vi "WaveformDAQ_tb2.vi"() -> ()   [LabVIEW 2018]
uses:
  <vilib>/DAQmx/read.llb/DAQmx Read (Analog Wfm 1Chan NSamp).vi
  <vilib>/DAQmx/create/channels.llb/DAQmx Create Channel (AI-Voltage-Basic).vi
  <vilib>/DAQmx/configure/timing.llb/DAQmx Timing (Sample Clock).vi
  <vilib>/DAQmx/miscellaneous.llb/DAQmx Fill In Error Info.vi
  <instrlib>/Agilent 33XXX Series/Agilent 33XXX Series.lvlib
  <resource>/objmgr/daqmx.rc
panel:
  out "Waveform Graph 2":waveform(dbl)(graph)
  in  "Sample Clock Source":tag="OnboardClock"
  out "error out":errorcluster
  out "Actual Sample Rate":dbl=1000.0 format="%0.2f"
  in  "Sample Mode":i32(ring)=10123 items=["Finite Samples"=10178, "Continuous Samples"=10123, "Hardware Timed Single Point"=12522]
  in  "Terminal Configuration":i32(ring)=-1 items=["default"=-1, "RSE"=10083, "NRSE"=10078, "Differential"=10106, "Pseudodifferential"=12529]
  in  "Voltage Max Value":dbl=5.0 caption="Max Value"
  in  "Voltage Min Value":dbl=-5.0 caption="Min Value"
  in  "Voltage Physical Channels":tag="Dev1/ai0" caption="Physical Channels"
  in  "stop":bool
  out "Waveform Graph":waveform(dbl)(graph)
  in  "Amplitude (1 Vpp)":dbl=1.0
  in  "DC Offset (0.00 V)":dbl
  in  "Waveform Function (1: Sine)":u16(ring)=1 items=["DC", "Sine", "Square", "Triangle", "Ramp", "Pulse", "Noise", "Sinc", "Negative Ramp", "Exponential Rise", "Exponential Fall", "Cardiac"]
  in  "Frequency (1000 Hz)":dbl=1000.0
  in  "Sample rate":enum16{"1KHz", "10KHz", "100KHz", "1MHz"}(ring)
  in  "Time":dbl
  out "N Samples":dbl
  in  "Serial Configuration":T1={"Baud Rate"=9600, "Parity"=0, "Data Bits"=8, "Flow Control"=4} {"Flow Control" items=["None", "XON/XOFF", "RTS/CTS", "XON/XOFF & RTS/CTS", "DTR/DSR", "XON/XOFF & DTR/DSR"]; "Data Bits" items=["7"=7, "8"=8]; "Parity" items=["None", "Odd", "Even", "Mark", "Space"]; "Baud Rate" items=["300"=300, "600"=600, "1200"=1200, "2400"=2400, "4800"=4800, "9600"=9600, "19200"=19200]}
  in  "VISA resource name":refnum<visa-resource-name>
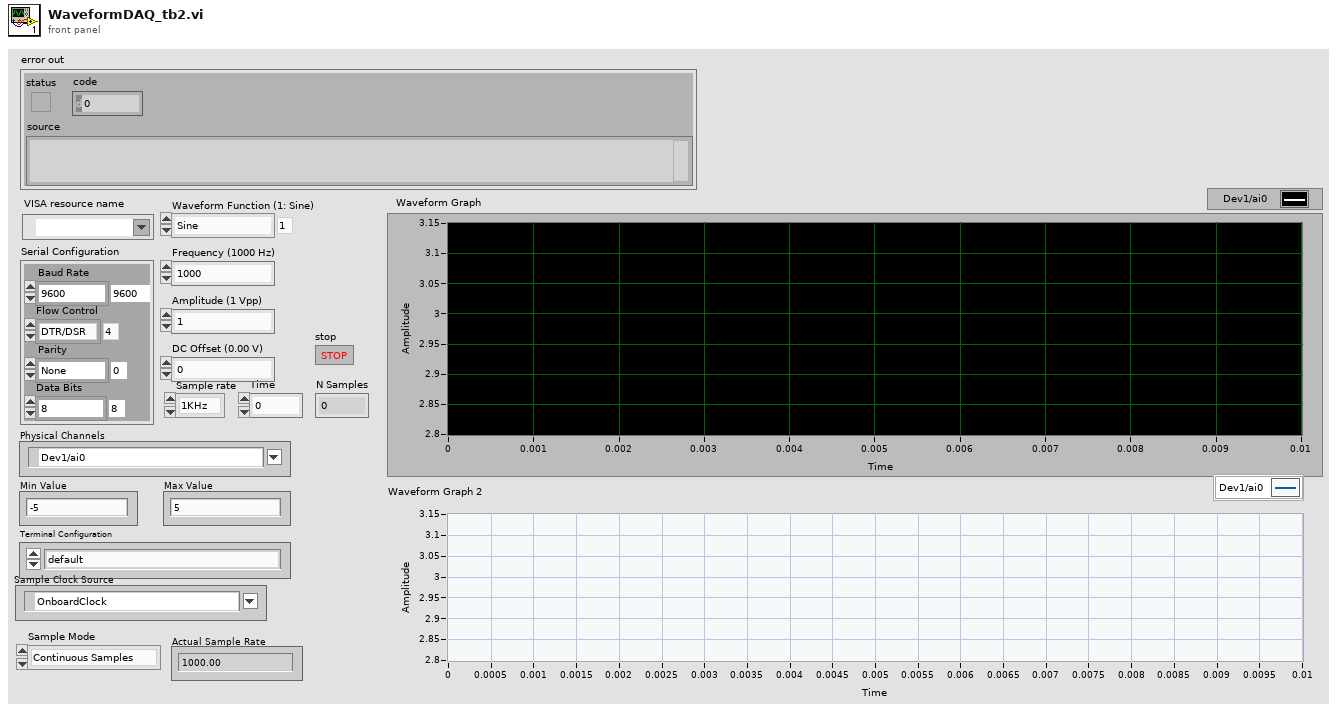
[diagram p1: front panel]
types:
  T1 = cluster{"Baud Rate":u32, "Parity":u16, "Data Bits":u16, "Flow Control":u16}
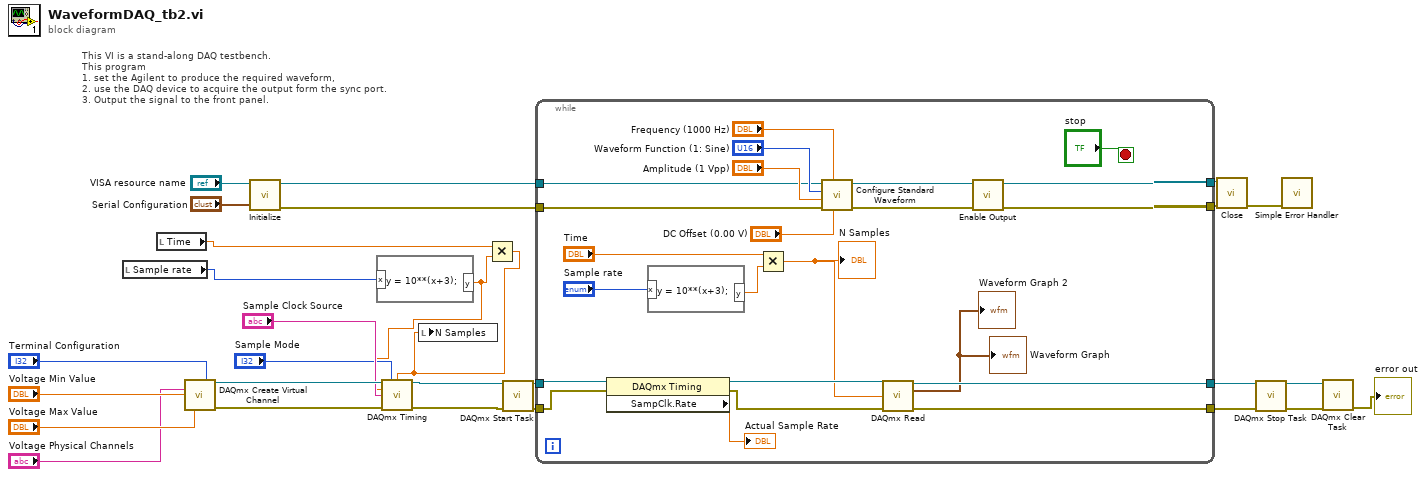
[diagram p0: block diagram]
diagram:
  # "This VI is a stand-along DAQ testbench.  \nThis program \n1. set the Agilent to produce the required waveform,\n2. use the DAQ device to acquire the output form the sync port. \n3. Output the signal to the front panel."
  n1 = local read "Sample rate"() -> (w1:enum16{"1KHz", "10KHz", "100KHz", "1MHz"})
  n2 = local read "Time"() -> (w2:dbl)
  n3 = call-poly <vilib>:"DAQmx Create Virtual Channel.vi"("maximum value"="Voltage Max Value", "minimum value"="Voltage Min Value", "input terminal configuration"="Terminal Configuration", "physical channels"="Voltage Physical Channels") -> ("task out"=w8:refnum<k21>, "error out"=w9:errorcluster)  [unwired: 10 in]
  n4 = call <instrlib>:"Initialize.vi"("Serial Configuration"="Serial Configuration", "VISA resource name"="VISA resource name") -> ("error out"=w23:errorcluster, "VISA resource name out"=w22:refnum<visa-resource-name>)  [unwired: 8 in]
  n5 = formula code="y = 10**(x+3);"("x"=w1) -> ("y"=w3:dbl)
  n6 = Multiply(x=w2, y=w3) -> (x*y=w4:dbl)
  n7 = call-poly <vilib>:"DAQmx Timing.vi"("task/channels in"=w8, "sample mode"="Sample Mode", "samples per channel"=w4, "rate"=w3, "source"="Sample Clock Source", "error in"=w9) -> ("task out"=w7:refnum<k21>, "error out"=w10:errorcluster)  [unwired: 8 in]
  n8 = local write "N Samples"(w4) -> ()
  n9 = call <vilib>:"DAQmx Start Task.vi"("task/channels in"=w7, "error in"=w10) -> ("task out"=w17:refnum<k21>, "error out"=w16:errorcluster)  [unwired: 12 in]
  n10 = while {
    tunnel: [w41] -> w25
    tunnel: [w42] -> w24
    tunnel: w23 -> [w44]
    tunnel: w22 -> [w43]
    tunnel: w17 -> [w34]
    tunnel: w16 -> [w33]
    tunnel: [w39] -> w15
    tunnel: [w38] -> w14
    stop <- "stop" stop-if-true
    n11 = property class="DAQmx Timing"(reference=w34, error in=w33) -> (reference out=w35:refnum<k21>, error out=w36:errorcluster, "SampClk.Rate"=→"Actual Sample Rate":dbl)
    n12 = formula code="y = 10**(x+3);"("x"="Sample rate") -> ("y"=w37:dbl)
    n13 = Multiply(x="Time", y=w37) -> (x*y=w32:dbl)
    "N Samples" <- w32
    n14 = call <instrlib>:"Configure Standard Waveform.vi"("DC Offset (0.00 V)"="DC Offset (0.00 V)", "Frequency (1000 Hz)"="Frequency (1000 Hz)", "error in (no error)"=w44, "Amplitude (1)"="Amplitude (1 Vpp)", "Waveform Function (1: Sine)"="Waveform Function (1: Sine)", "VISA resource name"=w43) -> ("error out"=w49:errorcluster, "VISA resource name out"=w48:refnum<visa-resource-name>)  [unwired: 4 in]
    n15 = call-poly <vilib>:"DAQmx Read.vi"("task/channels in"=w35, "number of samples per channel"=w32, "error in"=w36) -> ("task out"=w39:refnum<k21>, "data"=→"Waveform Graph" →"Waveform Graph 2":waveform(dbl), "error out"=w38:errorcluster)  [unwired: 10 in]
    n16 = call <instrlib>:"Enable Output.vi"("error in (no error)"=w49, "VISA resource name"=w48) -> ("error out"=w42:errorcluster, "VISA resource name out"=w41:refnum<visa-resource-name>)  [unwired: 8 in]
  }
  n17 = call <instrlib>:"Close.vi"("error in (no error)"=w24, "VISA resource name"=w25) -> ("error out"=w27:errorcluster)  [unwired: 9 in]
  n18 = call <vilib>:"DAQmx Stop Task.vi"("task/channels in"=w15, "error in"=w14) -> ("task out"=w13:refnum<k21>, "error out"=w12:errorcluster)  [unwired: 12 in]
  n19 = call <vilib>:"Simple Error Handler.vi"("error in (no error)"=w27) -> ()  [unwired: 4 in, 5 out]
  n20 = call <vilib>:"DAQmx Clear Task.vi"("task in"=w13, "error in"=w12) -> ("error out"=→"error out":errorcluster)  [unwired: 13 in]
